vi "pixel_XY_to_1D_index.vi"(1 "Y":i32, 2 "X":i32, 3 "Image Height":i32) -> (0 "ID Index":i32)   [LabVIEW 2019]
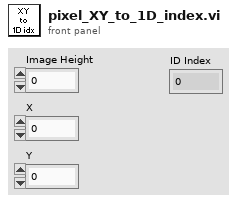
[diagram p1: front panel]
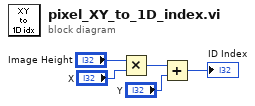
[diagram p0: block diagram]
diagram:
  n1 = Multiply(x="Image Height", y="X") -> (x*y=w5:i32)
  n2 = Add(x=w5, y="Y") -> (x+y=→"ID Index":i32)
